vi "Timelapse window-Initialise globals.vi"   [LabVIEW 2013]
uses:
  Globals/gl_Time series viewer globals.vi
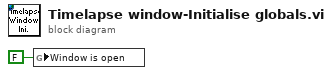
[diagram p0: block diagram]
diagram:
  n1 = global write "gl_Time series viewer globals.vi" "Window is open"(FALSE ("Bring to front")) -> ()
